vi "EMG_DESC_main.vi"() -> ()   [LabVIEW 2023]
doc: "This VI is the main VI for the EMG DESC Project, where is possible to set the main parameters. Indeed, it is possible to set the file path, select the desired EMG signal (between raw and envelopped), define the cutoff frequencies of the filters, and the thresholds for the EMG segmentation.\nMoreover it allows the visualisation of the Preprocessed signals, the main steps of the processed ones and to adjust at runtime the thresholds for further analysis."
panel:
  in  "Relative path":enum16{"Data\\DESC.csv", "Data/DESC.csv"}(ring)
  in  "Type of Signal":enum16{"Raw", "Envelopped"}(ring)
  out "Error Detector":errorcluster
  out "Raw imported signal":waveform(dbl)(graph)
  in  "Raw Highpass cutoff freq [Hz]":dbl=20.0 format="%0.4f"
  in  "Raw Lowpass cutoff freq [Hz]":dbl=200.0
  in  "Raw Stop":bool
  out "Raw Processed over Threshold":waveform(dbl)(graph)
  in  "Raw Threshold":dbl(slide)=0.5 min=0.0 max=1.0 scale=0.0..1.0
  out "Raw Filtered":waveform(dbl)(graph)
  out "Raw Filtered + Rectified + Normalised":waveform(dbl)(graph)
  out "Envelopped imported signal":waveform(dbl)(graph)
  in  "Env. Lowpass cutoff freq [Hz]":dbl=200.0
  in  "Envelopped Threshold":dbl(slide)=0.5 min=0.0 max=1.0 scale=0.0..1.0
  out "Env Processed over Threshold":waveform(dbl)(graph)
  in  "Env Stop":bool
  out "Envelopped Filtered + Normalised":waveform(dbl)(graph)
  in  "Acquired Samping Frequency [Hz]":dbl=2000.0
  out "Headers Data":string[](array[string])
  out "Data [V]":dbl[][](array[numeric])
  out "Complete Path":path
  # "EMG DESC ELECTRODES"
  # "Data Import"
  # "Data Visualisation"
  # "Data Processing"
  # "Data Thresholding"
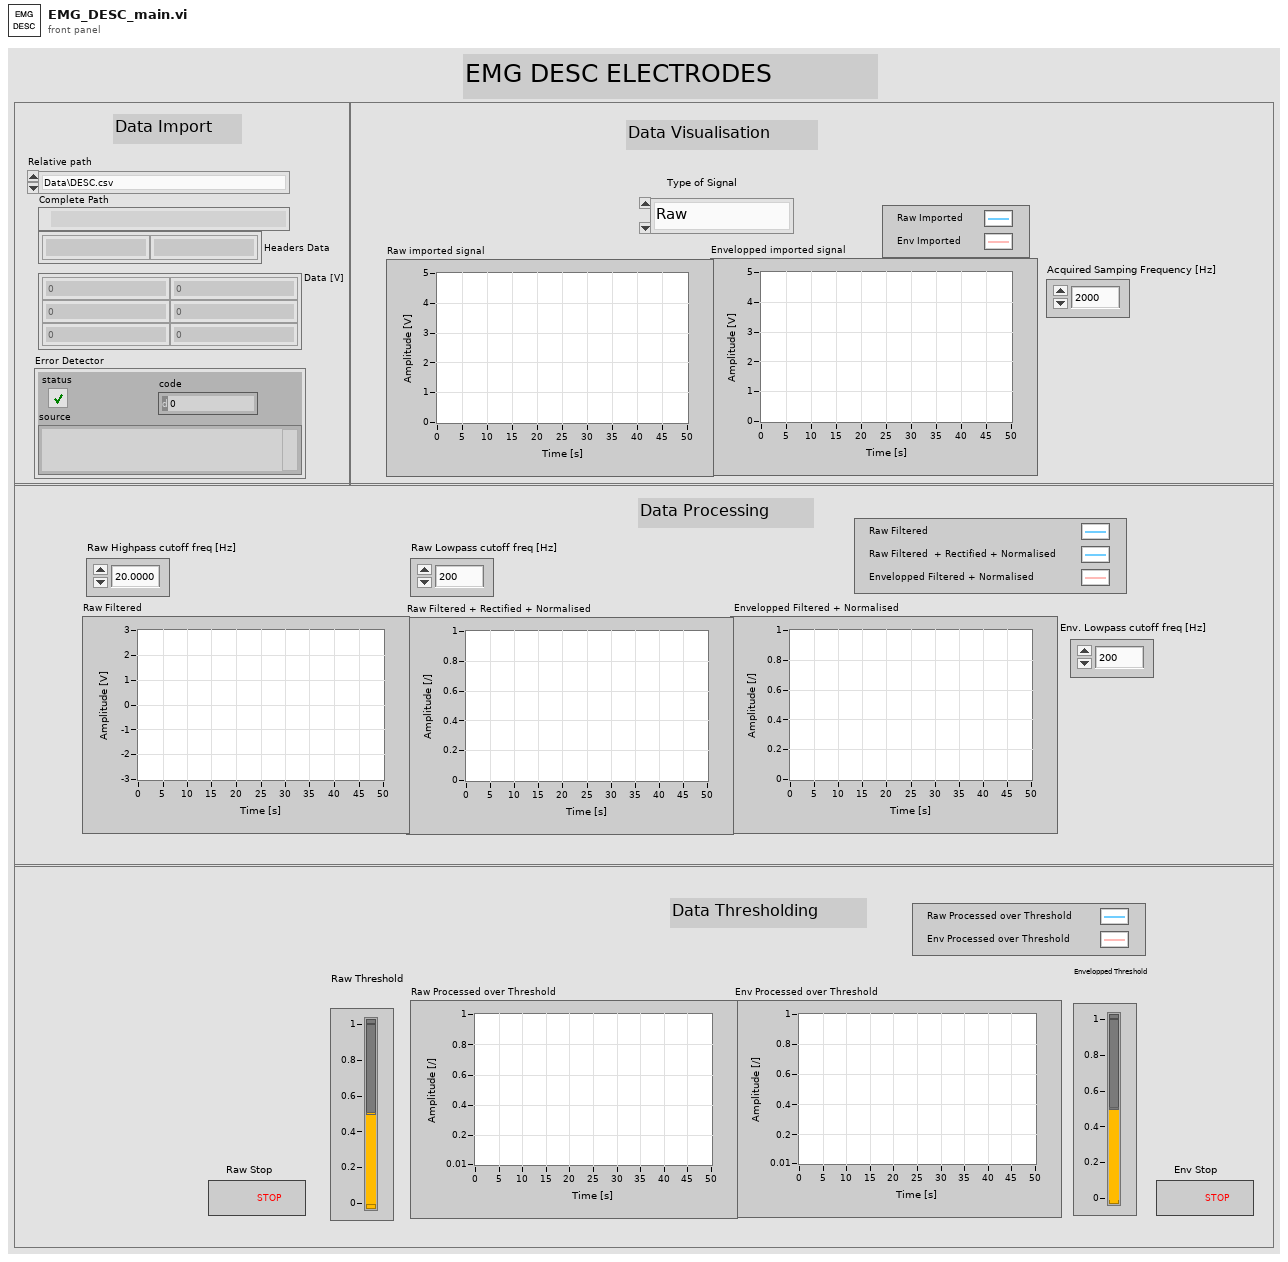
[diagram p1: front panel]
types:
  T1 = cluster{"Data Output [V]":dbl[][], "Type of Signal":enum16{"Raw", "Envelopped"}}
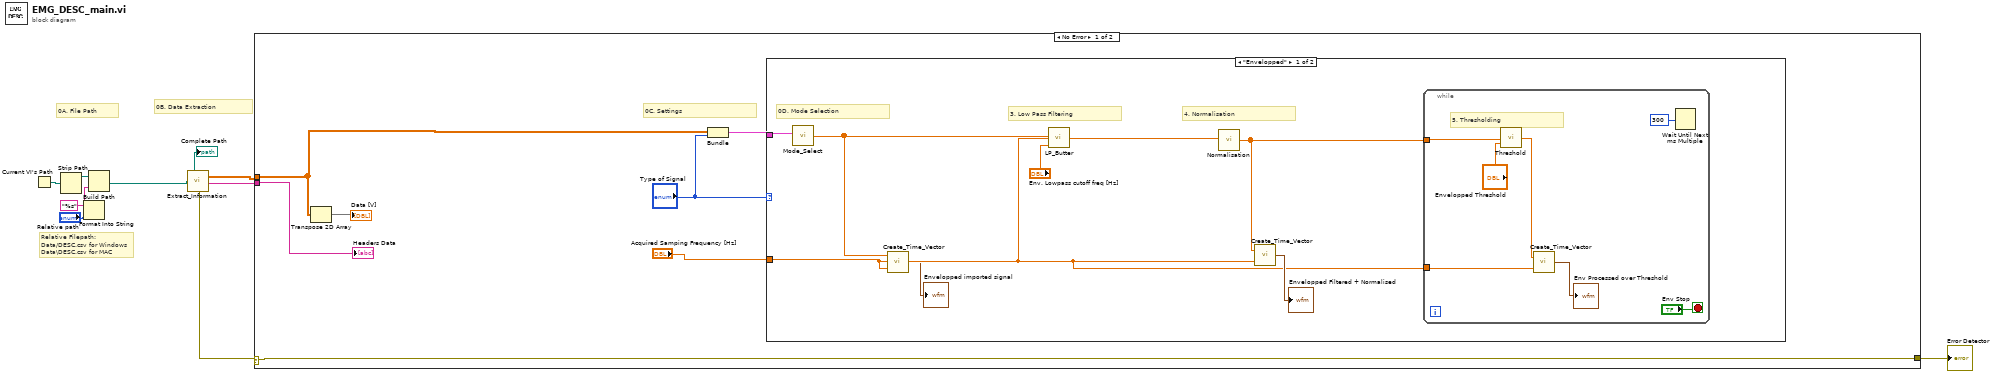
[diagram p0: block diagram]
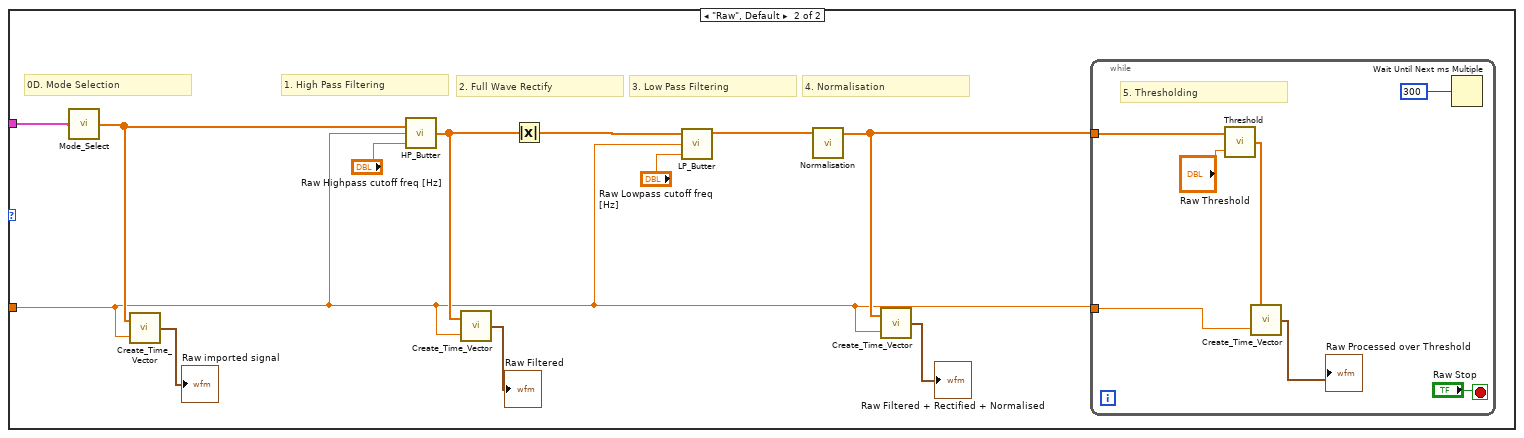
[diagram p2: hidden frame]
diagram:
  # "0B. Data Extraction"
  # "Relative Filepath:\nData/DESC.csv for Windows\nData\\DESC.csv for MAC"
  # "0A. File Path"
  n1 = Current VI's Path() -> (path=w11:path)
  n2 = Strip Path(path=w11) -> (stripped path=w10:path)  [unwired: 1 out]
  n3 = Format Into String(format string="%s", "Relative path") -> (resulting string=w1:string)  [unwired: 2 in, 1 out]
  n4 = Build Path(base path=w10, name or relative path=w1) -> (appended path=w7:path)
  n5 = call "Extract_Information.vi"("Input Path"=w7) -> ("File path (Not A Path if cancelled)"=→"Complete Path":path, "Headers"=w5:string[], "Data Output [V]"=w6:dbl[][], "Error on importing Data"=w8:errorcluster)
  n6 = case shown="No Error" w8 {
    selector: w8 -> [w13 w53]
    tunnel: w6 -> [w15 _]
    tunnel: w5 -> [w14 _]
    tunnel: [w13 w53] -> w9
    frame No Error {
      # "0C. Settings"
      n7 = Transpose 2D Array(2D array=w15) -> (transposed array=→"Data [V]":dbl[][])
      n8 = Bundle("Data Output [V]"=w15, "Type of Signal"="Type of Signal") -> (w18:T1)  [unwired: 1 in]
      n9 = case shown="\"Envelopped\"" "Type of Signal" {
        tunnel: w18 -> [w22 w37]
        tunnel: "Acquired Samping Frequency [Hz]" -> [w20 w35]
        frame "Envelopped" {
          # "4. Normalisation"
          # "3. Low Pass Filtering"
          # "0D. Mode Selection"
          n10 = call "Mode_Select.vi"("Input Data"=w22) -> ("Signal Sequence [V]"=w21:dbl[])
          n11 = call "Create_Time_Vector.vi"("Samping Frequency [Hz]"=w20, "Data Vector [V]"=w21) -> ("Waveform"=→"Envelopped imported signal":waveform(dbl))
          n12 = call "LP_Butter.vi"("Low cutoff freq [Hz]"="Env. Lowpass cutoff freq [Hz]", "Samping Frequency [Hz]"=w20, "Signal Sequence [V]"=w21) -> ("Low Pass Filtered Data [V]"=w25:dbl[])
          n13 = call "Normalisation.vi"("Input Time Serie [V]"=w25) -> ("Normalised Time Serie [\\]"=w24:dbl[])
          n14 = call "Create_Time_Vector.vi"("Samping Frequency [Hz]"=w20, "Data Vector [V]"=w24) -> ("Waveform"=→"Envelopped Filtered + Normalised":waveform(dbl))
          n15 = while {
            tunnel: w24 -> [w32]
            tunnel: w20 -> [w30]
            stop <- "Env Stop" stop-if-true
            # "5. Thresholding"
            n16 = call "Threshold.vi"("Threshold"="Envelopped Threshold", "Normalised Time Serie [\\]"=w32) -> ("Thresholded Time Serie [\\]"=w31:dbl[])
            n17 = call "Create_Time_Vector.vi"("Samping Frequency [Hz]"=w30, "Data Vector [V]"=w31) -> ("Waveform"=→"Env Processed over Threshold":waveform(dbl))
            n18 = Wait Until Next ms Multiple(millisecond multiple=u32 300) -> ()  [unwired: 1 out]
          }
        }
        frame "Raw", Default {
          # "4. Normalisation"
          # "3. Low Pass Filtering"
          # "2. Full Wave Rectify"
          # "1. High Pass Filtering"
          # "0D. Mode Selection"
          n19 = call "Mode_Select.vi"("Input Data"=w37) -> ("Signal Sequence [V]"=w36:dbl[])
          n20 = call "Create_Time_Vector.vi"("Samping Frequency [Hz]"=w35, "Data Vector [V]"=w36) -> ("Waveform"=→"Raw imported signal":waveform(dbl))
          n21 = call "HP_Butter.vi"("Highpass cutoff freq [Hz]"="Raw Highpass cutoff freq [Hz]", "Samping Frequency [Hz]"=w35, "Signal Sequence [V]"=w36) -> ("High Pass Filtered Data [V]"=w44:dbl[])
          n22 = call "Create_Time_Vector.vi"("Samping Frequency [Hz]"=w35, "Data Vector [V]"=w44) -> ("Waveform"=→"Raw Filtered":waveform(dbl))
          n23 = Absolute Value(x=w44) -> (abs(x)=w43:dbl[])
          n24 = call "LP_Butter.vi"("Low cutoff freq [Hz]"="Raw Lowpass cutoff freq [Hz]", "Samping Frequency [Hz]"=w35, "Signal Sequence [V]"=w43) -> ("Low Pass Filtered Data [V]"=w42:dbl[])
          n25 = call "Normalisation.vi"("Input Time Serie [V]"=w42) -> ("Normalised Time Serie [\\]"=w40:dbl[])
          n26 = call "Create_Time_Vector.vi"("Samping Frequency [Hz]"=w35, "Data Vector [V]"=w40) -> ("Waveform"=→"Raw Filtered + Rectified + Normalised":waveform(dbl))
          n27 = while {
            tunnel: w40 -> [w52]
            tunnel: w35 -> [w51]
            stop <- "Raw Stop" stop-if-true
            # "5. Thresholding"
            n28 = call "Threshold.vi"("Threshold"="Raw Threshold", "Normalised Time Serie [\\]"=w52) -> ("Thresholded Time Serie [\\]"=w50:dbl[])
            n29 = call "Create_Time_Vector.vi"("Samping Frequency [Hz]"=w51, "Data Vector [V]"=w50) -> ("Waveform"=→"Raw Processed over Threshold":waveform(dbl))
            n30 = Wait Until Next ms Multiple(millisecond multiple=u32 300) -> ()  [unwired: 1 out]
          }
        }
      }
      "Headers Data" <- w14
    }
    frame Error, Default {
    }
  }
  "Error Detector" <- w9
